vi "Get Signals.vi"(8 "error in (no error)":errorcluster, 10 "Connection String":string) -> (0 "error out":errorcluster, 2 "Array":string[](array[string]))   [LabVIEW 2022 SP3]
doc: "This example demonstrates how to list both visible and invisible signals of a device."
uses:
  <instrlib>/openDAQ/Public/Classes/IInstance/IInstance.lvclass
  C:/Program Files (x86)/National Instruments/LabVIEW 2022/instr.lib/openDAQ/Public/Classes/IDevice/IDevice.lvclass
  <instrlib>/openDAQ/Public/Classes/ISignal/ISignal.lvclass
  C:/Program Files (x86)/National Instruments/LabVIEW 2022/instr.lib/openDAQ/Public/Classes/IComponent/IComponent.lvclass
  <instrlib>/openDAQ/Public/Classes/IDevice/IDevice.lvclass
  <instrlib>/openDAQ/Public/Classes/daqUtils/daqUtils.lvlib
  <instrlib>/openDAQ/Public/Classes/IComponent/IComponent.lvclass
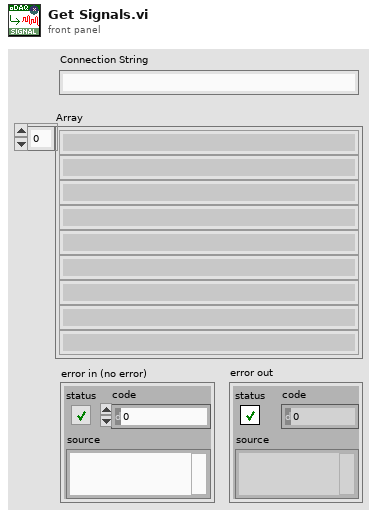
[diagram p1: front panel]
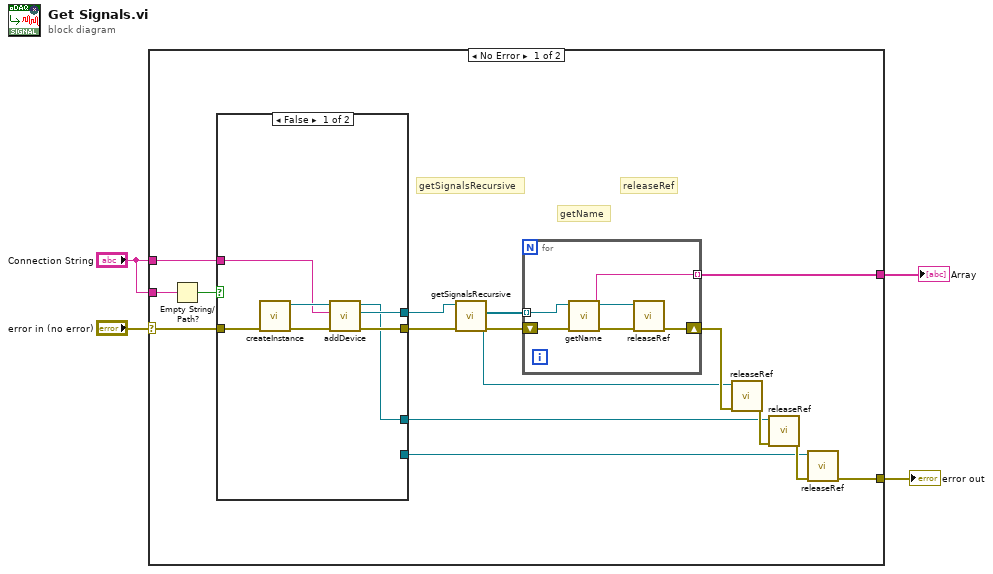
[diagram p0: block diagram]
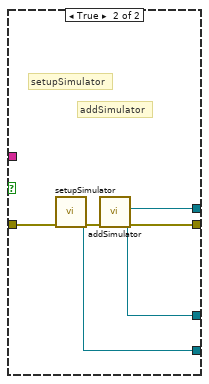
[diagram p2: hidden frame]
diagram:
  n1 = case shown="No Error" "error in (no error)" {
    selector: "error in (no error)" -> [w6 w40]
    tunnel: [w15 _] -> w4
    tunnel: [w11 w40] -> w3
    tunnel: "Connection String" -> [w8 _]
    tunnel: "Connection String" -> [w5 _]
    frame No Error {
      # "releaseRef"
      # "getName"
      # "getSignalsRecursive"
      n2 = Empty String/Path?(string/path=w8) -> (empty?=w7:bool)
      n3 = case shown="False" w7 {
        tunnel: w6 -> [w25 w33]
        tunnel: [w24 w31] -> w18
        tunnel: [w21 w30] -> w13
        tunnel: [_ w29] -> w10
        tunnel: [w22 w28] -> w9
        tunnel: w5 -> [w23 _]
        frame False {
          n4 = call <instrlib>:"createInstance.vi"("error in (no error)"=w25) -> ("error out"=w27:errorcluster, "IInstance out"=w26:refnum<class "IInstance.lvclass">)  [unwired: 9 in]
          n5 = call <instrlib>:"addDevice.vi"("error in (no error)"=w27, "ConnectionString in"=w23, "IDevice in"=w26) -> ("error out"=w24:errorcluster, "ConnectedDevice out"=w22:refnum<class "IDevice.lvclass">, "IDevice out"=w21:refnum<class "IInstance.lvclass">)  [unwired: 6 in]
        }
        frame True {
          # "addSimulator"
          # "setupSimulator"
          n6 = call <instrlib>:"setupSimulator.vi"("error in (no error)"=w33) -> ("error out"=w32:errorcluster, "IInstance out"=w29:refnum<class "IInstance.lvclass">)  [unwired: 9 in]
          n7 = call <instrlib>:"addSimulator.vi"("error in (no error)"=w32) -> ("error out"=w31:errorcluster, "IDevice out"=w28:refnum<class "IDevice.lvclass">, "IInstance out"=w30:refnum<class "IInstance.lvclass">)  [unwired: 8 in]
        }
      }
      n8 = call <instrlib>:"getSignalsRecursive.vi"("error in (no error)"=w18, "IDevice in"=w9) -> ("error out"=w16:errorcluster, "Available Sigals out"=w17:refnum<class "ISignal.lvclass">[], "IDevice out"=w14:refnum<class "IDevice.lvclass">)  [unwired: 7 in]
      n9 = for {
        tunnel: w17 -> [w38] mode=indexing
        shift-right: [w36] -> w20
        shift-left: w16 -> [w39]
        tunnel: [w34] -> w15 mode=indexing
        n10 = call <instrlib>:"getName.vi"("error in (no error)"=w39, "IComponent in"=w38) -> ("error out"=w37:errorcluster, "Name out"=w34:string, "IComponent out"=w35:refnum<class "ISignal.lvclass">)  [unwired: 7 in]
        n11 = call-dynamic "releaseRef.vi"("error in (no error)"=w37, "IBaseObject in"=w35) -> ("error out"=w36:errorcluster)  [unwired: 9 in]
      }
      n12 = call-dynamic "releaseRef.vi"("error in (no error)"=w20, "IBaseObject in"=w14) -> ("error out"=w19:errorcluster)  [unwired: 9 in]
      n13 = call-dynamic "releaseRef.vi"("error in (no error)"=w19, "IBaseObject in"=w13) -> ("error out"=w12:errorcluster)  [unwired: 9 in]
      n14 = call-dynamic "releaseRef.vi"("error in (no error)"=w12, "IBaseObject in"=w10) -> ("error out"=w11:errorcluster)  [unwired: 9 in]
    }
    frame Error {
    }
  }
  "error out" <- w3
  "Array" <- w4
